vi "Destroy Events.vi"(8 "error in":errorcluster) -> (0 "error out":errorcluster)   [LabVIEW 2020]
doc: "Destroy all user events.\n\n-----\nJuan Navarro\nLab it Studio"
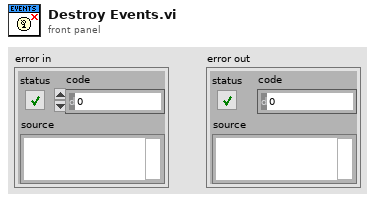
[diagram p1: front panel]
types:
  T1 = enum16{"Create Event", "Generate Event", "Destroy Event"}
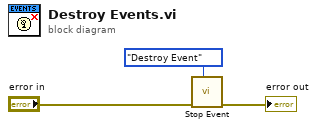
[diagram p0: block diagram]
diagram:
  n1 = call "Stop Event.vi"("Actions"=T1."Destroy Event", "error in"="error in") -> ("error out"=→"error out":errorcluster)  [unwired: 8 in, 1 out]
